vi "CRYReport Frame.vi"() -> ()   [LabVIEW 2013]
uses:
  CRYReport Global.vi
panel:
  in  "nIDV":i32
  in  "StateOut":bool
  in  "nIDF":i32
  in  "stop":bool
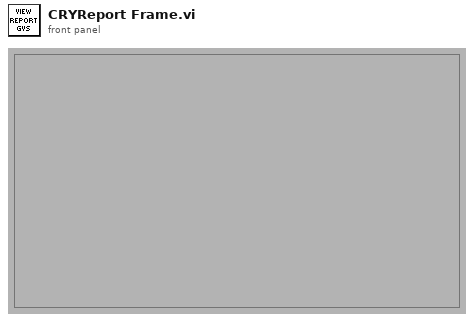
[diagram p1: front panel]
types:
  T1 = cluster{"sAction":string, "sType":string, "sQueueName":string, "sGraphName":string, "sData":string, "nData":i32, "pVIRef":refnum<vi>, "pSPRef":refnum<vi>}
  T2 = cluster{"nID":i16, "sName":string, "pVIRef":refnum<vi>, "pSPRef":refnum<vi>, "sTitle":string, "nIDObject":i16, "nIDV":i16, "nWidth":i16, "nHeight":i16, "bImgChange":bool, "sType":string, "sState":string, "sPosition":string, "sData":string}
  T3 = cluster{"nID":i32, "sName":string, "sType":string, "sProperty":string, "sTemplet":string, "sDocking":string, "pVIRef":refnum<vi>, "pSPRef":refnum<vi>, "pRefTemplet":refnum<vi>, "pRefSplitter":refnum<vi>[], "nPosSplitter":i32[], "pRefSP":refnum<vi>[], "nSPID":i32[], "sSPDock":string[], "nIDFrame":i32[], "nIDPanel":i32[], "nActiveFrame":i32, "nCountFrame":i32, "cFrame":cluster{"nID":i32, "sName":string, "sType":string, "sTitle":string, "sIcon":string, "pVIRef":refnum<vi>, "pSPRef":refnum<vi>, "cWiin":cluster{"sName":string, "sType":string, "pVIRef":refnum<vi>, "sData":string}, "cTab":cluster{"sTitle":string, "sIcon":string, "pSpliter":refnum<vi>, "nAvtivePage":i32, "nIDPage":i32[], "nIDFrame":i32[]}, "sData":string}[], "sData":string, "sSplitterName":string[]}
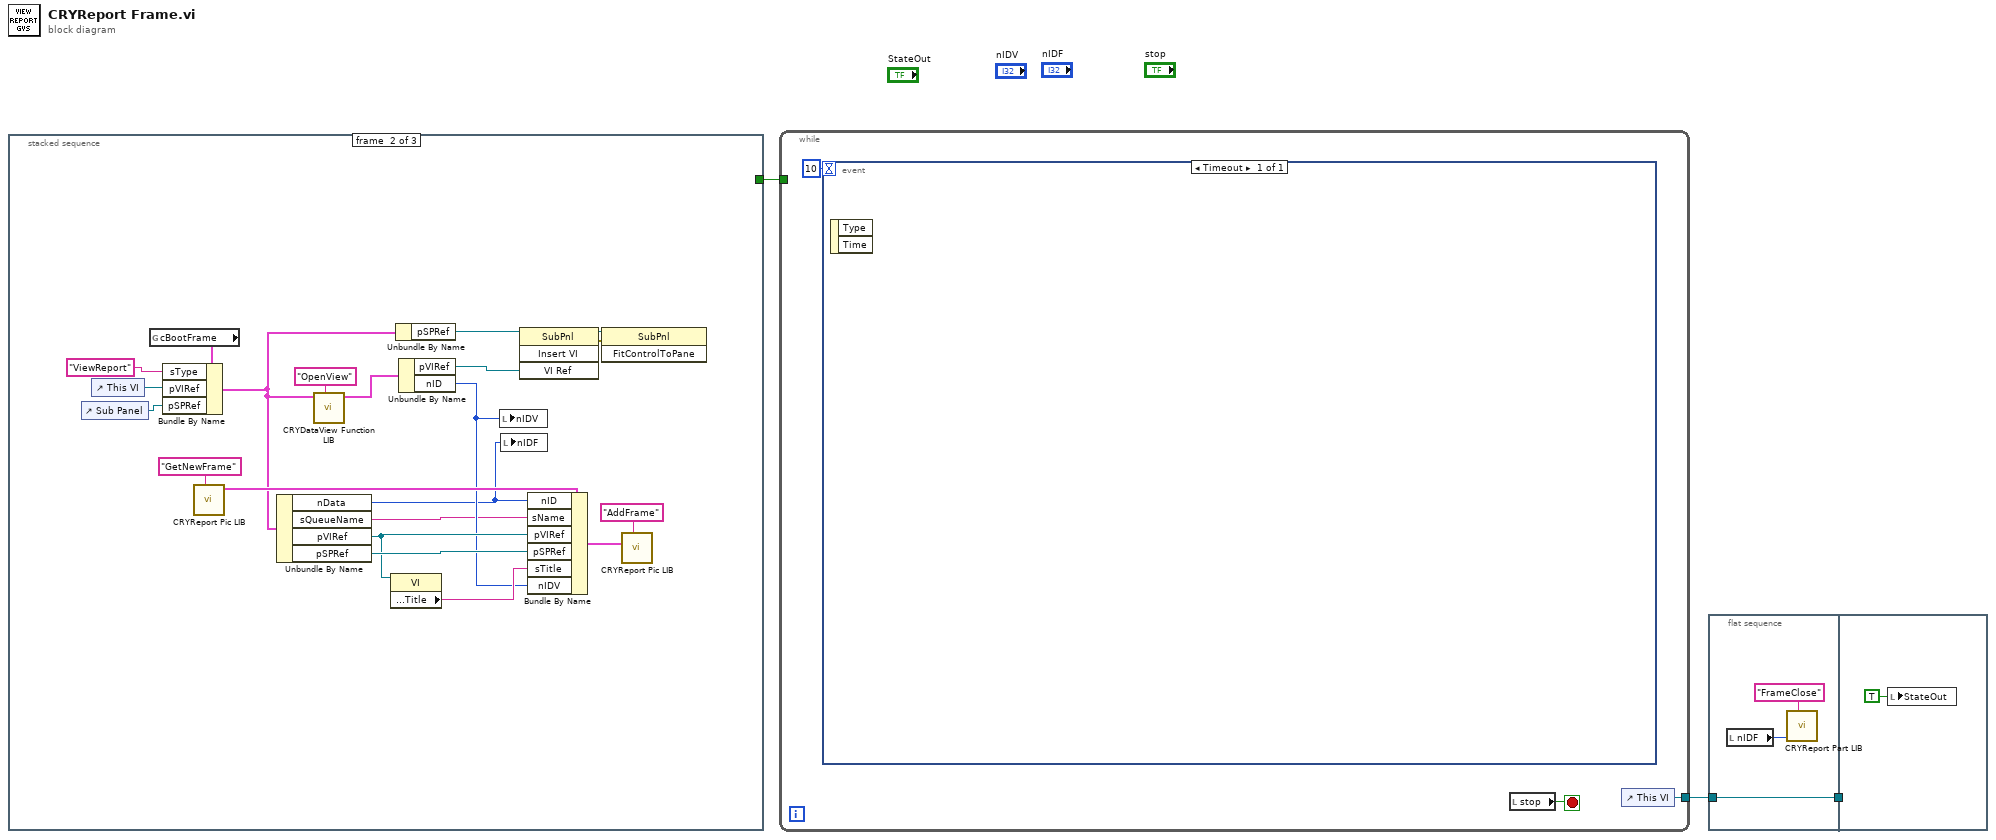
[diagram p0: block diagram]
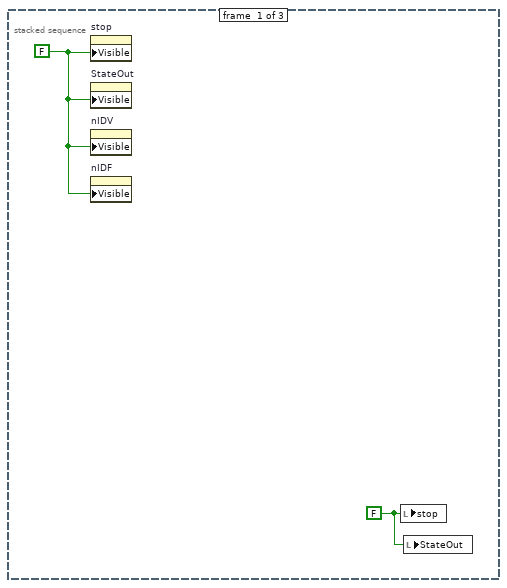
[diagram p2: hidden frame]
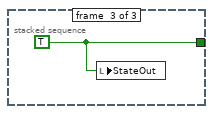
[diagram p3: hidden frame]
diagram:
  n1 = stacked-sequence {
    tunnel: [_ _ w27] -> w3
    frame #0 {
      w5 = FALSE ("stop")
      w4 = FALSE ("Visible")
      n2 = property on="stop" class="Bool (strict)"("Visible"=w4) -> ()  [unwired: 2 in, 2 out]
      n3 = property on="StateOut" class="Bool (strict)"("Visible"=w4) -> ()  [unwired: 2 in, 2 out]
      n4 = property on="nIDV" class="DigNum (strict)"("Visible"=w4) -> ()  [unwired: 2 in, 2 out]
      n5 = property on="nIDF" class="DigNum (strict)"("Visible"=w4) -> ()  [unwired: 2 in, 2 out]
      n6 = local write "stop"(w5) -> ()
      n7 = local write "StateOut"(w5) -> ()
    }
    frame #1 {
      n8 = control-ref of="Sub Panel"() -> (w23:refnum<vi>)
      n9 = control-ref of="This VI"() -> (w22:refnum<vi>)
      n10 = global read "CRYReport Global.vi" "cBootFrame"() -> (w24:T1)
      n11 = Bundle By Name(cluster=w24, "sType"="ViewReport", "pVIRef"=w22, "pSPRef"=w23) -> (w19:T1)
      n12 = call "CRYReport Pic LIB.vi"("sAction"="GetNewFrame") -> ("cFrame_Out"=w20:T2)  [unwired: 7 in, 3 out]
      n13 = Unbundle By Name(w19) -> ("nData"=w11:i32, "sQueueName"=w12:string, "pVIRef"=w17:refnum<vi>, "pSPRef"=w18:refnum<vi>)
      n14 = call "CRYDataView Function LIB.vi"("sAction"="OpenView", "cBootVIEW"=w19) -> ("cView_Out"=w7:T3)  [unwired: 7 in, 2 out]
      n15 = property class="VI"(reference=w17) -> ("Front Panel.Title"=w16:string)  [unwired: 1 in, 2 out]
      n16 = Unbundle By Name(w19) -> ("pSPRef"=w26:refnum<vi>)
      n17 = Unbundle By Name(w7) -> ("pVIRef"=w10:refnum<vi>, "nID"=w15:i32)
      n18 = local write "nIDV"(w15) -> ()
      n19 = local write "nIDF"(w11) -> ()
      n20 = invoke class="SubPnl" method="Insert VI"(reference=w26, "VI Ref"=w10) -> (reference out=w8:refnum<vi>, error out=w9:errorcluster)  [unwired: 2 in, 2 out]
      n21 = Bundle By Name(cluster=w20, "nID"=w11, "sName"=w12, "pVIRef"=w17, "pSPRef"=w18, "sTitle"=w16, "nIDV"=w15) -> (w14:T2)
      n22 = invoke class="SubPnl" method="FitControlToPane"(reference=w8, error in=w9) -> ()  [unwired: 1 in, 3 out]
      n23 = call "CRYReport Pic LIB.vi"("sAction"="AddFrame", "cFrame"=w14) -> ()  [unwired: 6 in, 4 out]
    }
    frame #2 {
      w27 = TRUE ("StateOut")
      n24 = local write "StateOut"(w27) -> ()
    }
  }
  n25 = while {
    tunnel: w3 -> [_]
    tunnel: [w28] -> w1
    stop <- w30 stop-if-true
    n26 = event shown="[0] Timeout" {
      selector: _ -> [_]
      dyn-events: _ -> [_]
      timeout: 10 -> [_]
      event Timeout {
        n27 = event-data() -> ()  [unwired: 1 in, 2 out]
      }
    }
    n28 = local read "stop"() -> (w30:bool)
    n29 = control-ref of="This VI"() -> (w28:refnum<vi>)
  }
  n30 = flat-sequence {
    tunnel: [w33] -> w2
    tunnel: w1 -> [w33]
    tunnel: w2 -> [_]
    frame #0 {
      n31 = local read "nIDF"() -> (w32:i32)
      n32 = call "CRYReport Part LIB.vi"("sAction"="FrameClose", "nData"=w32) -> ()  [unwired: 6 in, 4 out]
    }
    frame #1 {
      n33 = local write "StateOut"(TRUE ("StateOut")) -> ()
    }
  }
